vi "LinearFilter_LowPassBW2.vi"(9 "SamplePeriod":dbl format="%13.5p", 11 "TimeConstant":dbl format="%13.5p") -> (3 "LINEAR_FILTER":T1 {"Outputs" format="%13.5g"; "Inputs" format="%13.5g"; "OutputGains" format="%13.5g"; "InputGains" format="%13.5g"})   [LabVIEW 2019, in "Trajectory_Library.lvlib"]
doc: "Creates a 2nd order Butterworth low pass filter.\n\nA 2nd order filter provides more filtering, however it also has a larger phase shift (time delay).\n\nMore information on this type of filter can be found at:\n\n https://en.wikipedia.org/wiki/Butterworth_filter\n\nInputs: \n - timeConstant - The discrete-time time constant in seconds.\n - samplePeriod - The period in seconds between samples taken by the user.\n\nOutputs:\n - Linearfilter - Created datat structure"
uses:
  Trajectory_Library.lvlib
  TypeDef/LINEAR_FILTER.ctl
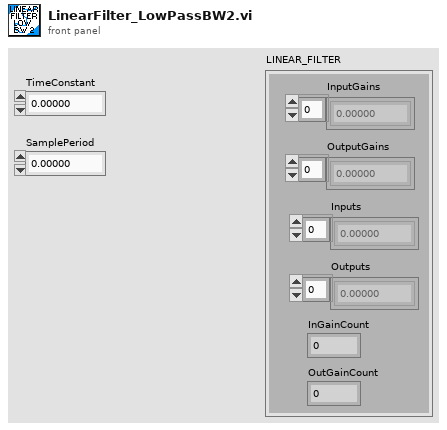
[diagram p1: front panel]
types:
  T1 = typedef "Trajectory_Library.lvlib/LINEAR_FILTER.ctl" = cluster{"InputGains":dbl[], "OutputGains":dbl[], "Inputs":dbl[], "Outputs":dbl[], "InGainCount":i32, "OutGainCount":i32}
  T2 = typedef "WPILib_Math.lvlib/LINEAR_FILTER.ctl" = cluster{"InputGains":dbl[], "OutputGains":dbl[], "Inputs":dbl[], "Outputs":dbl[], "InGainCount":i32, "OutGainCount":i32}
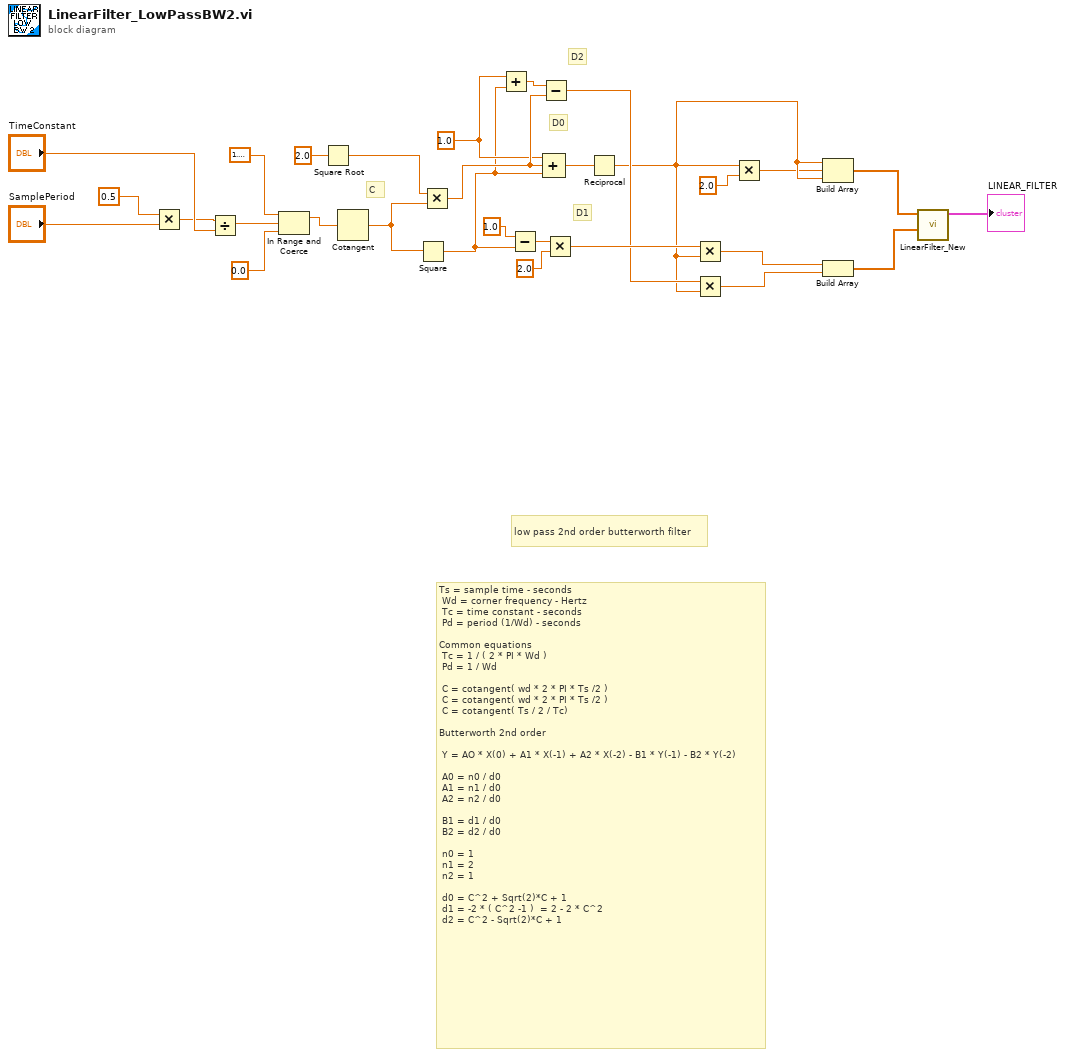
[diagram p0: block diagram]
diagram:
  w14 = 1.0 ("value")
  # "D2"
  # "D1"
  # "D0"
  # "Ts = sample time - seconds\n\tWd = corner frequency - Hertz\n\tTc = time constant - seconds\n\tPd = period (1/Wd) - seconds\n\nCommon equations\n\tTc = 1 / ( 2 * PI * Wd )\n\tPd = 1 / Wd\n\t\n\tC = cotangent( wd * 2 * PI * Ts /2 )\n C = cotangent( wd * 2 * PI * Ts /2 )\n C = cotangent( Ts / 2 / Tc)\n\nButterworth 2nd order\n\n\tY = AO * X(0) + A1 * X(-1) + A2 * X(-2) - B1 * Y(-1) - B2 * Y(-2)\n\n\tA0 = n0 / d0\n\tA1 = n1 / d0\n\tA2 = n2 / d0\n\n\tB1 = d1 / d0\n\tB2 = d2 / d0\n\n\tn0 = 1\n\tn1 = 2\n\tn2 = 1\n\n\td0 = C^2 + Sqrt(2)*C + 1\n\td1 = -2 * ( C^2 -1 )  = 2 - 2 * C^2\n\td2 = C^2 - Sqrt(2)*C + 1"
  # "C"
  # "low pass 2nd order butterworth filter"
  n1 = Multiply(x=0.5, y="SamplePeriod") -> (x*y=w24:dbl)
  n2 = Divide(x=w24, y="TimeConstant") -> (x/y=w2:dbl)
  n3 = In Range and Coerce(upper limit=1.5707963267948966, x=w2, lower limit=0.0) -> (coerced(x)=w1:dbl)  [unwired: 1 out]
  n4 = Square Root(x=2.0) -> (sqrt(x)=w21:dbl)
  n5 = Cotangent(1:w1) -> (0:w20:dbl)
  n6 = Square(x=w20) -> (x^2=w13:dbl)
  n7 = Multiply(x=w21, y=w20) -> (x*y=w15:dbl)
  n8 = Add(x=w14, y=w13) -> (x+y=w16:dbl)
  n9 = Subtract(x=1.0 ("y"), y=w13) -> (x-y=w19:dbl)
  n10 = Subtract(x=w16, y=w15) -> (x-y=w10:dbl)
  n11 = Compound Arithmetic op=ADD(w14, w15, w13) -> (w12:dbl)
  n12 = Multiply(x=w19, y=2.0) -> (x*y=w11:dbl)
  n13 = Reciprocal(x=w12) -> (1/x=w6:dbl)
  n14 = Multiply(x=w11, y=w6) -> (x*y=w9:dbl)
  n15 = Multiply(x=w10, y=w6) -> (x*y=w8:dbl)
  n16 = Multiply(x=w6, y=2.0) -> (x*y=w5:dbl)
  n17 = Build Array(w6, w5, w6) -> (w29:dbl[])
  n18 = Build Array(w9, w8) -> (w27:dbl[])
  n19 = call "LinearFilter_New.vi"("OutputGains"=w27, "InputGains"=w29) -> ("LINEAR_FILTER"=→"LINEAR_FILTER":T2)  [unwired: 9 in]
